vi "Range.vi"() -> ()   [LabVIEW 2013]
panel:
  in  "Range":dbl
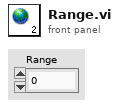
[diagram p1: front panel]
diagram:
